vi "Decode Inverter State.vi"(11 "Byte In":u8) -> (3 "Inverter State Out":T1)   [LabVIEW 2014]
uses:
  Inverter States.ctl
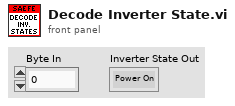
[diagram p1: front panel]
types:
  T1 = typedef "Inverter States.ctl" = enum16{"Power On", "Stop", "Open Loop", "Closed Loop", "Wait", "Internal", "Idle Run", "Idle Stop", ""}
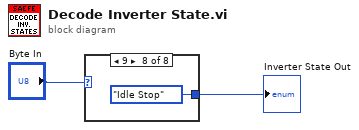
[diagram p0: block diagram]
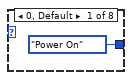
[diagram p2: hidden frame]
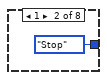
[diagram p3: hidden frame]
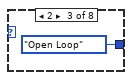
[diagram p4: hidden frame]
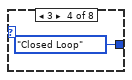
[diagram p5: hidden frame]
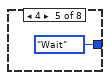
[diagram p6: hidden frame]
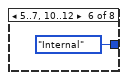
[diagram p7: hidden frame]
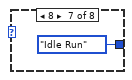
[diagram p8: hidden frame]
diagram:
  n1 = case shown="9" "Byte In" {
    tunnel: [Inverter_States."Power On" ("Inverter") Inverter_States."Stop" ("Inverter") Inverter_States."Open Loop" ("Inverter") Inverter_States."Closed Loop" ("Inverter") Inverter_States."Wait" ("Inverter") Inverter_States."Internal" ("Inverter") Inverter_States."Idle Run" ("Inverter") Inverter_States."Idle Stop" ("Inverter")] -> w2
    frame 0, Default {
    }
    frame 1 {
    }
    frame 2 {
    }
    frame 3 {
    }
    frame 4 {
    }
    frame 5..7, 10..12 {
    }
    frame 8 {
    }
    frame 9 {
    }
  }
  "Inverter State Out" <- w2
